vi "Generic Camera Wait For New Frame Ref Timeout.vi"(0 "Image Ref":T1, 2 "Timeout (ms)":u32=1000, 11 "Error In":errorcluster, 13 "Wait No. (1)":u32=1) -> (4 "Image Ref Out":T1, 15 "Error Out":errorcluster)   [LabVIEW 2025]
uses:
  <vilib>/vision/Image Controls.llb/IMAQ Image.ctl
  Camera Controls/Camera IMAQ Key Info.ctl
panel:
  out "Timed Out":bool
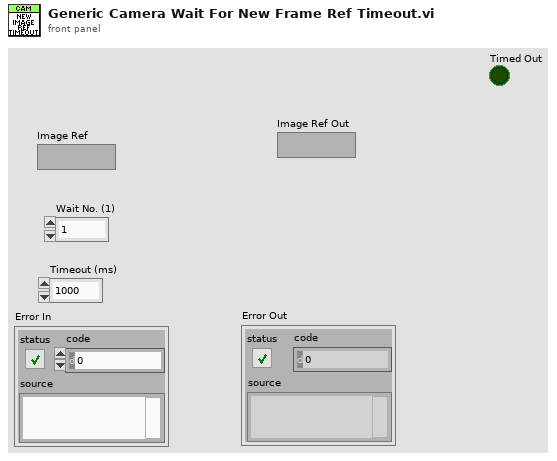
[diagram p1: front panel]
types:
  T1 = typedef "IMAQ Image.ctl" = refnum<image>
  T2 = typedef "Camera IMAQ Key Info.ctl" = cluster{"Frame":u32, "Sensor Height":i32, "Sensor Width":i32, "ROI Height":i32, "ROI Width":i32, "ROI Enable?":bool, "Bit per Pixel":u8}
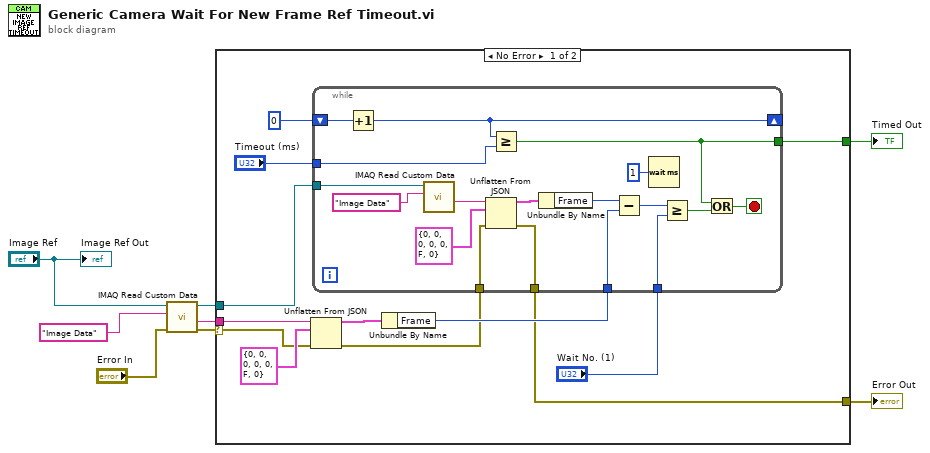
[diagram p0: block diagram]
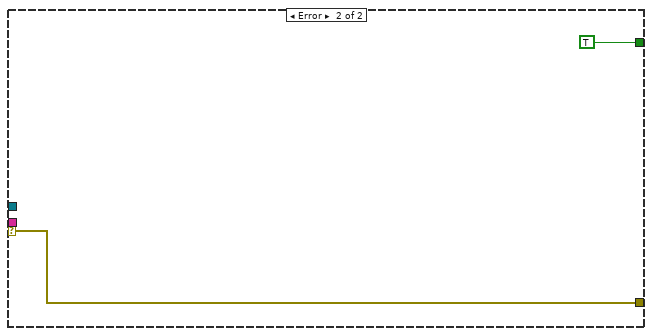
[diagram p2: hidden frame]
diagram:
  n1 = call "IMAQ Read Custom Data"("error in (no error)"="Error In", "Key"="Image Data", "Image"="Image Ref") -> ("error out"=w5:errorcluster, "Custom Data Out"=w8:string, "Image (duplicate)"=w6:T1)  [unwired: 6 in]
  n2 = case shown="No Error" w5 {
    selector: w5 -> [w14 w40]
    tunnel: w8 -> [w18 _]
    tunnel: w6 -> [w17 _]
    tunnel: [w12 w40] -> w2
    tunnel: [w9 TRUE] -> w1
    frame No Error {
      n3 = Unflatten From JSON(JSON string=w18, type and defaults=T2 {"Frame"=0, "Sensor Height"=0, "Sensor Width"=0, "ROI Height"=0, "ROI Width"=0, "ROI Enable?"=FALSE, "Bit per Pixel"=0} ("Camera IMAQ Key Info"), error in (no error)=w14) -> (value=w20:T2, error out=w13:errorcluster)  [unwired: 4 in]
      n4 = Unbundle By Name(w20) -> ("Frame"=w16:u32)
      n5 = while {
        tunnel: w17 -> [w34]
        tunnel: w16 -> [w32]
        tunnel: "Wait No. (1)" -> [w30]
        tunnel: w13 -> [w29]
        tunnel: [w28] -> w12
        shift-right: [w25] -> _
        shift-left: u32 0 -> [w27]
        tunnel: "Timeout (ms)" -> [w26]
        tunnel: [w21] -> w9
        stop <- w22 stop-if-true
        n6 = Increment(x=w27) -> (x+1=w25:u32)
        n7 = call "IMAQ Read Custom Data"("Key"="Image Data", "Image"=w34) -> ("Custom Data Out"=w36:string)  [unwired: 7 in, 2 out]
        n8 = Unflatten From JSON(JSON string=w36, type and defaults=T2 {"Frame"=0, "Sensor Height"=0, "Sensor Width"=0, "ROI Height"=0, "ROI Width"=0, "ROI Enable?"=FALSE, "Bit per Pixel"=0} ("Camera IMAQ Key Info"), error in (no error)=w29) -> (value=w38:T2, error out=w28:errorcluster)  [unwired: 4 in]
        n9 = Greater Or Equal?(x=w25, y=w26) -> (x >= y?=w21:bool)
        n10 = Unbundle By Name(w38) -> ("Frame"=w33:u32)
        n11 = Subtract(x=w33, y=w32) -> (x-y=w31:u32)
        n12 = Wait (ms)(milliseconds to wait=u32 1) -> ()  [unwired: 1 out]
        n13 = Greater Or Equal?(x=w31, y=w30) -> (x >= y?=w23:bool)
        n14 = Or(x=w21, y=w23) -> (x .or. y?=w22:bool)
      }
    }
    frame Error {
    }
  }
  "Error Out" <- w2
  "Timed Out" <- w1
  "Image Ref Out" <- "Image Ref"
